vi "INSERT.vi"(6 "Time Stamp":timestamp, 8 "error in":errorcluster, 9 "Data":variant, 10 "Path(s)":variant, 11 "Data.PG in":refnum<class "LV-Data.PGSQL.lvclass">) -> (0 "error out":errorcluster, 1 "Wrote to DB?":bool, 2 "Paths out":string, 3 "Data.PG out":refnum<class "LV-Data.PGSQL.lvclass">)   [LabVIEW 2019, in "LV-Data.PGSQL.lvclass"]
uses:
  LV-Data.PGSQL.lvclass
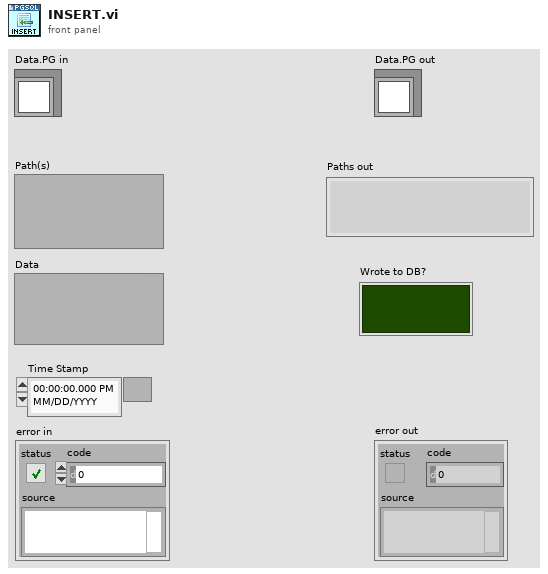
[diagram p1: front panel]
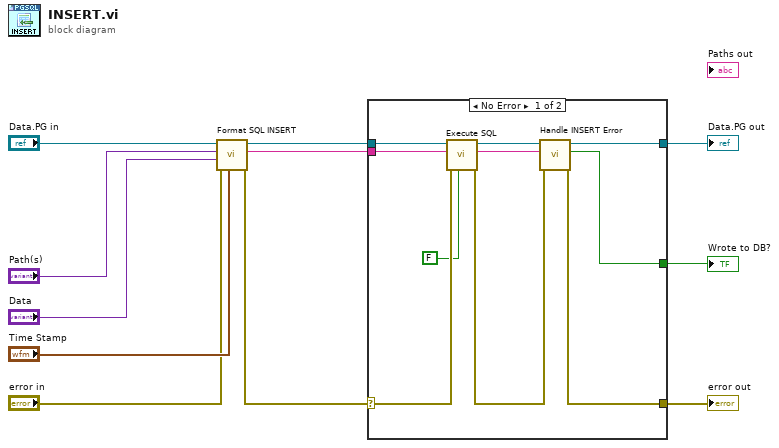
[diagram p0: block diagram]
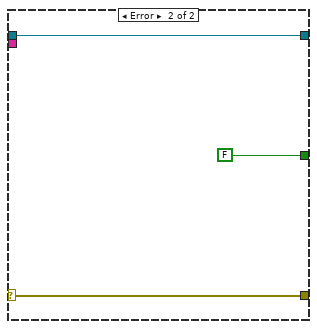
[diagram p2: hidden frame]
diagram:
  n1 = call "Format SQL INSERT.vi"("Time Stamp"="Time Stamp", "error in"="error in", "Data"="Data", "Path(s)"="Path(s)", "LV-Data.PGSQL in"="Data.PG in") -> ("error out"=w8:errorcluster, "Formatted Insert"=w9:string, "LV-Data.PGSQL out"=w1:refnum<class "LV-Data.PGSQL.lvclass">)  [unwired: 3 in, 1 out]
  n2 = case shown="No Error" w8 {
    selector: w8 -> [w16 w22]
    tunnel: [w15 w22] -> w7
    tunnel: w1 -> [w19 w24]
    tunnel: [w21 w24] -> w6
    tunnel: [w20 FALSE] -> w11
    tunnel: w9 -> [w13 _]
    frame No Error {
      n3 = call "Execute SQL.vi"("Result?"=FALSE, "error in"=w16, "SQL"=w13, "LV-Data.PGSQL"=w19) -> ("error out"=w17:errorcluster, "SQL out"=w12:string, "LV-Data.PGSQL out"=w18:refnum<class "LV-Data.PGSQL.lvclass">)  [unwired: 4 in, 1 out]
      n4 = call "Handle INSERT Error.vi"("error in (no error)"=w17, "SQL"=w12, "Database.PG"=w18) -> ("error out"=w15:errorcluster, "Wrote to DB?"=w20:bool, "Database.PG out"=w21:refnum<class "LV-Data.PGSQL.lvclass">)  [unwired: 6 in]
    }
    frame Error {
    }
  }
  "error out" <- w7
  "Data.PG out" <- w6
  "Wrote to DB?" <- w11
